vi "NewSerialDialog.vi"() -> (17 "执行完毕":bool)   [LabVIEW 2019]
uses:
  00 Ctl/SerialData.ctl
  02 Mode/SerialMode/SerialClass.lvclass
panel:
  in  "取消":bool
  in  "确认":bool
  in  "停止":bool
  in  "串口配置":T1={"VISA串口名称"="", "波特率"=9600, "停止位"=10, "流控制"=0, "数据位"=8, "奇偶校验"=enum."None", "超时"=2000, "启用终止符？"=FALSE, "终止符"=10} {"终止符" format="%.0x"; "数据位" min=5 max=8 step=1; "流控制" items=["无", "XON/XOFF", "RTS/CTS", "XON/XOFF & RTS/CTS", "DTR/DSR", "XON/XOFF & DTR/DSR"]; "停止位" items=["1.0"=10, "1.5"=15, "2.0"=20]; "波特率" items=["9600"=9600, "115200"=15]}
  # "用于控制数据流\n控制顺序"
  # "输出增加个有效判断\n区分取消和失败操作"
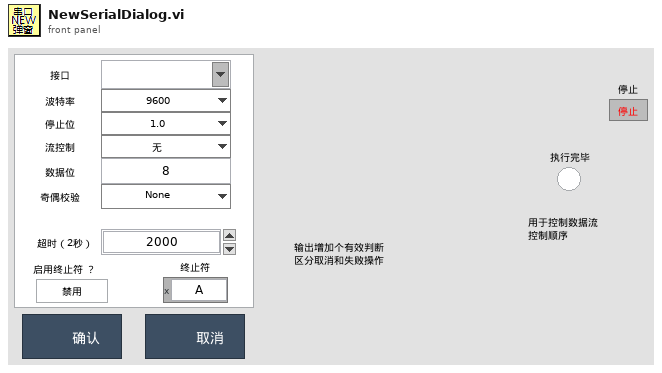
[diagram p1: front panel]
types:
  T1 = typedef "SerialData.ctl" = cluster{"VISA串口名称":refnum<visa-resource-name>, "波特率":u32, "停止位":u16, "流控制":u16, "数据位":u16, "奇偶校验":enum16{"None", "Odd", "Even", "Mark", "Space"}, "超时":u32, "启用终止符？":bool, "终止符":u8}
  T2 = typedef "串口枚举.ctl" = enum16{"ini", "增", "删", "查", "改"}
  T3 = cluster{"串口名称":string, "SerialClass 输出":refnum<class "SerialClass.lvclass">}
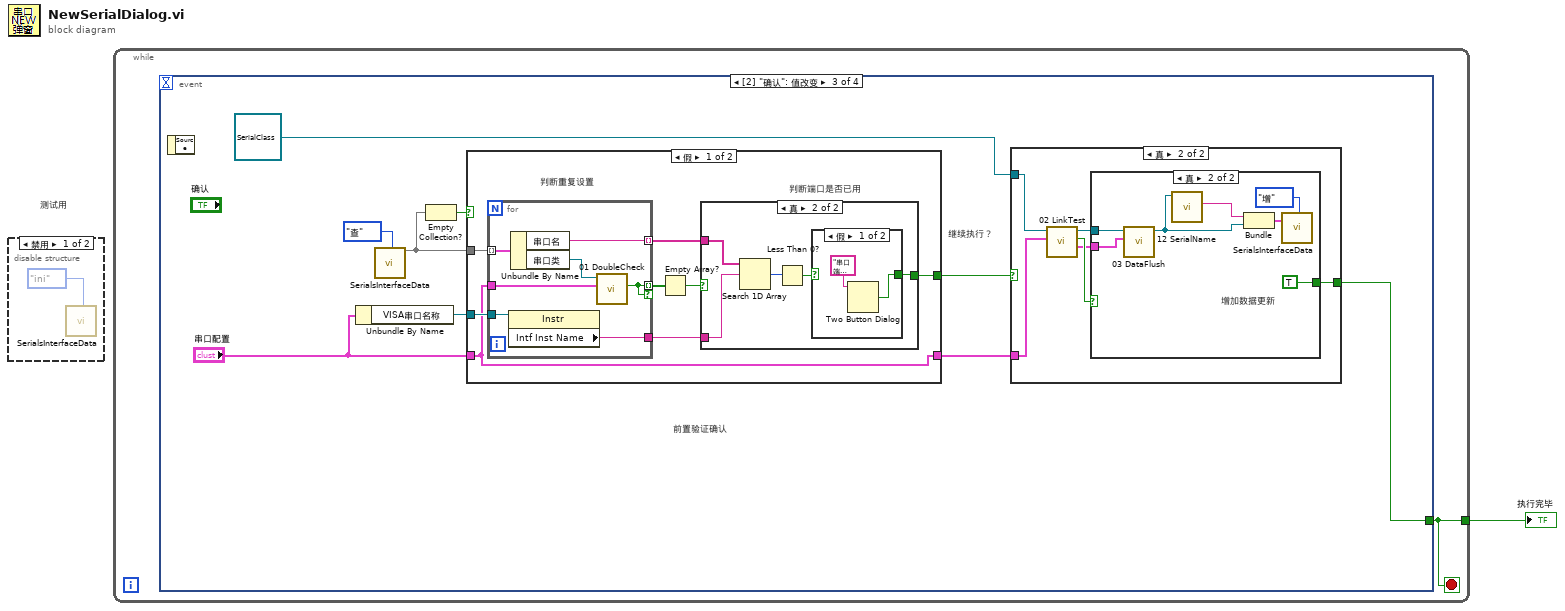
[diagram p0: block diagram]
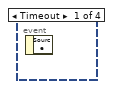
[diagram p3: hidden frame]
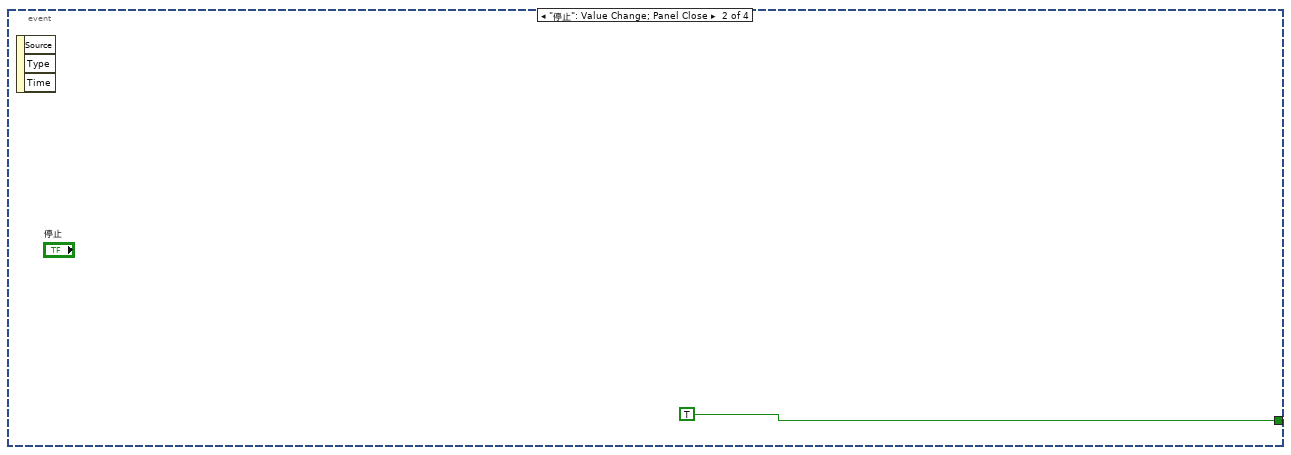
[diagram p4: hidden frame]
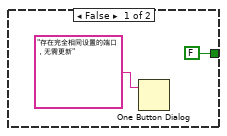
[diagram p7: hidden frame]
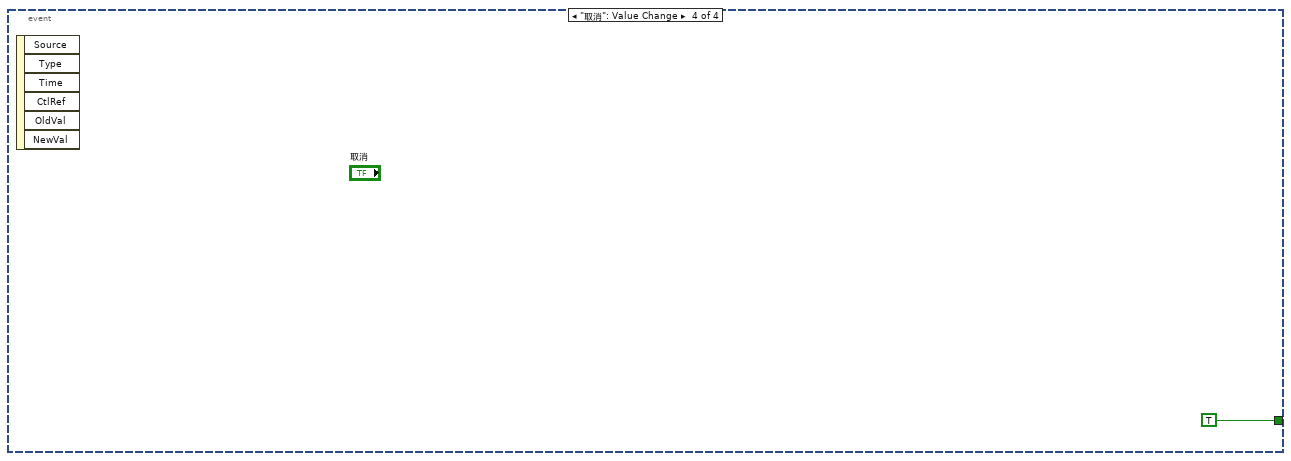
[diagram p10: hidden frame]
diagram:
  # "测试用"
  n1 = disable-structure shown="禁用" {
    frame Disabled {
      n2 = call "SerialsInterfaceData.vi"("串口枚举"=串口枚举."ini") -> ()  [unwired: 17 in, 2 out]
    }
    frame Enabled {
    }
  }
  n3 = while {
    tunnel: [w3] -> w1
    stop <- w3 stop-if-true
    n4 = event shown="[2] \"确认\": 值改变" {
      selector: _ -> [_ _ _ _]
      dyn-events: _ -> [_ _ _ _]
      timeout: _ -> [_ _ _ _]
      tunnel: [_ TRUE ("停止") w13 TRUE ("停止")] -> w3
      event Timeout {
        n5 = event-data() -> ()  [unwired: 1 in, 1 out]
      }
      event "停止": Value Change; Panel Close {
        n6 = event-data() -> ()  [unwired: 1 in, 3 out]
      }
      event "确认": Value Change {
        # "前置验证确认"
        # "继续执行？"
        n7 = event-data() -> ()  [unwired: 1 in, 1 out]
        n8 = Unbundle By Name("串口配置") -> ("VISA串口名称"=w9:refnum<visa-resource-name>)
        n9 = call "SerialsInterfaceData.vi"("串口枚举"=串口枚举."查") -> ("串口表"=w10:map{string, refnum<class "SerialClass.lvclass">})  [unwired: 17 in, 1 out]
        n10 = Empty Collection?(1:w10) -> (0:w11:bool)
        n11 = case shown="假" w11 {
          selector: w11 -> [_ w53]
          tunnel: w10 -> [w34 _]
          tunnel: "串口配置" -> [w27 w52]
          tunnel: w9 -> [w33 _]
          tunnel: [w28 w53] -> w8
          tunnel: [w27 w52] -> w7
          frame False {
            # "判断端口是否已用"
            # "判断重复设置"
            n12 = for {
              tunnel: w34 -> [w51] mode=indexing
              tunnel: w27 -> [w50]
              tunnel: w33 -> [w48]
              tunnel: [w45] -> w32 mode=indexing if=w45
              tunnel: [w47] -> w30
              tunnel: [w46] -> w29 mode=indexing
              n13 = property class="Instr"(reference=w48) -> ("Intf Inst Name"=w47:string)  [unwired: 1 in, 2 out]
              n14 = Unbundle By Name(w51) -> ("串口名"=w46:string, "串口类"=w49:refnum<class "SerialClass.lvclass">)
              n15 = call-dynamic "01 DoubleCheck.vi"("串口配置"=w50, "SerialClass 输入"=w49) -> ("重复？"=w45:bool)  [unwired: 6 in, 3 out]
            }
            n16 = Empty Array?(array=w32) -> (empty?=w31:bool)
            n17 = case shown="真" w31 {
              tunnel: w30 -> [_ w40]
              tunnel: w29 -> [_ w41]
              tunnel: [FALSE w37] -> w28
              frame False {
                n18 = One Button Dialog(message="存在完全相同设置的端口，无需更新" ("消息")) -> ()  [unwired: 1 in, 1 out]
              }
              frame True {
                n19 = Search 1D Array(1D array=w41, element=w40) -> (index of element=w39:i32)  [unwired: 1 in]
                n20 = Less Than 0?(x=w39) -> (x < 0?=w38:bool)
                n21 = case shown="假" w38 {
                  selector: w38 -> [_ w44]
                  tunnel: [w42 w44] -> w37
                  frame False {
                    n22 = Two Button Dialog(message="串口端正在使用，更新配置？" ("消息")) -> (T button?=w42:bool)  [unwired: 2 in]
                  }
                  frame True {
                  }
                }
              }
            }
          }
          frame True {
            # "第一个记录，绿灯"
          }
        }
        n23 = case shown="真" w8 {
          tunnel: refnum<class "SerialClass.lvclass"> refnum ("SerialClass.lvclass") -> [_ w19]
          tunnel: w7 -> [_ w18]
          tunnel: [_ w14] -> w13
          frame False {
          }
          frame True {
            n24 = call-dynamic "02 LinkTest.vi"("串口配置"=w18, "SerialClass 输入"=w19) -> ("串口已配置"=w15:T1, "成功？"=w17:bool, "SerialClass 输出"=w16:refnum<class "SerialClass.lvclass">)  [unwired: 6 in, 1 out]
            n25 = case shown="真" w17 {
              tunnel: w16 -> [_ w25]
              tunnel: w15 -> [_ w26]
              tunnel: [_ TRUE] -> w14
              frame False {
              }
              frame True {
                # "增加数据更新"
                n26 = call-dynamic "03 DataFlush.vi"("串口配置"=w26, "SerialClass 输入"=w25) -> ("SerialClass 输出"=w20:refnum<class "SerialClass.lvclass">)  [unwired: 8 in, 1 out]
                n27 = call-dynamic "12 SerialName.vi"("SerialClass 输入"=w20) -> ("串口名称"=w24:string)  [unwired: 8 in, 2 out]
                n28 = Bundle("串口名称"=w24, "SerialClass 输出"=w20) -> (w23:T3)  [unwired: 1 in]
                n29 = call "SerialsInterfaceData.vi"("信息"=w23, "串口枚举"=串口枚举."增") -> ()  [unwired: 16 in, 2 out]
              }
            }
          }
        }
      }
      event "取消": Value Change {
        n30 = event-data() -> ()  [unwired: 1 in, 6 out]
      }
    }
  }
  "执行完毕" <- w1
